vi "Test ADC command testing.vi"(8 "error in (no error)":errorcluster, 11 "TestCase in":refnum<class "Test ADC command.lvclass">) -> (0 "error out":errorcluster, 3 "TestCase out":refnum<class "Test ADC command.lvclass">)   [LabVIEW 2020, in "Test ADC command.lvclass"]
uses:
  Test ADC command.lvclass
  Implementation/Simulated Device/Simulated Device.lvclass
  <vilib>/addons/_JKI Toolkits/VI Tester/TestCase.llb/TestCase.lvclass
  C:/Program Files (x86)/National Instruments/LabVIEW 2020/vi.lib/addons/_JKI Toolkits/VI Tester/TestCase.llb/TestCase.lvclass
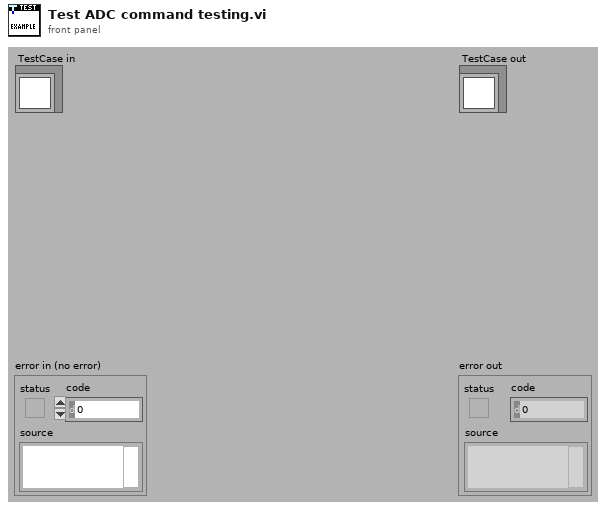
[diagram p1: front panel]
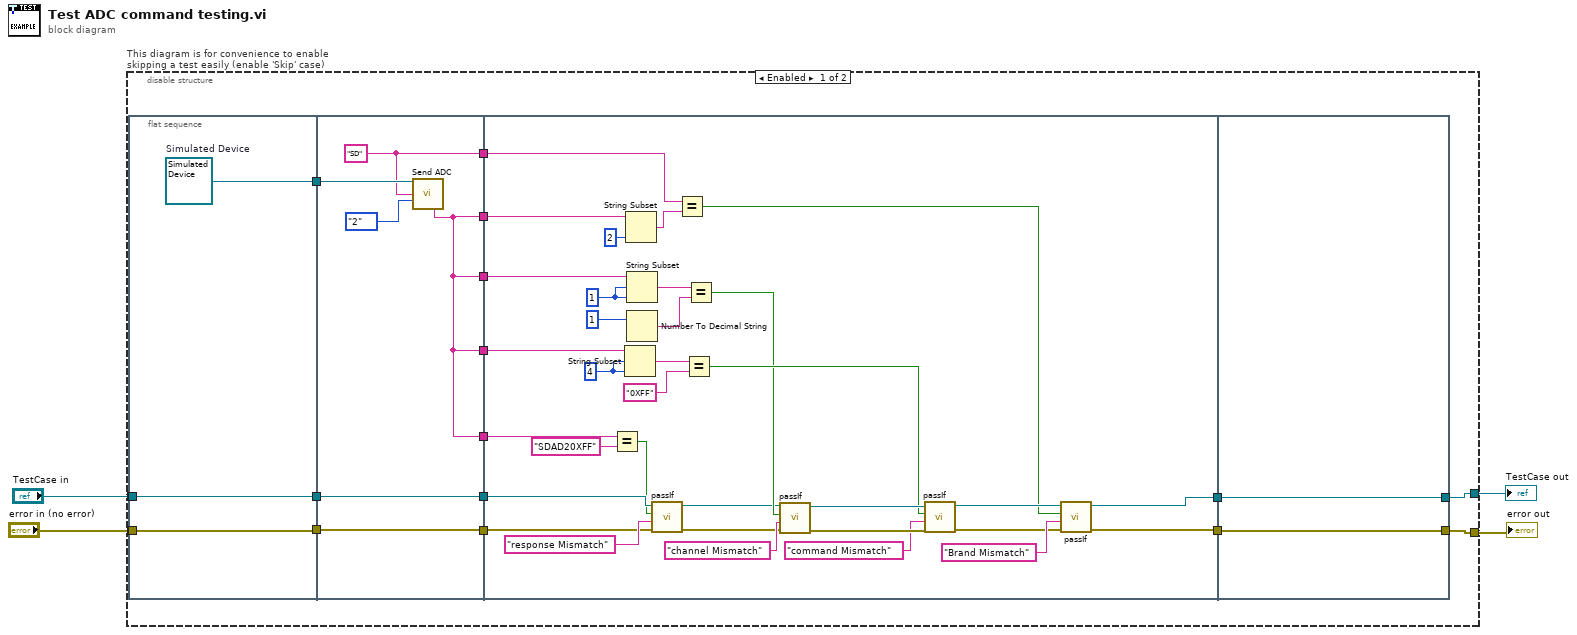
[diagram p0: block diagram]
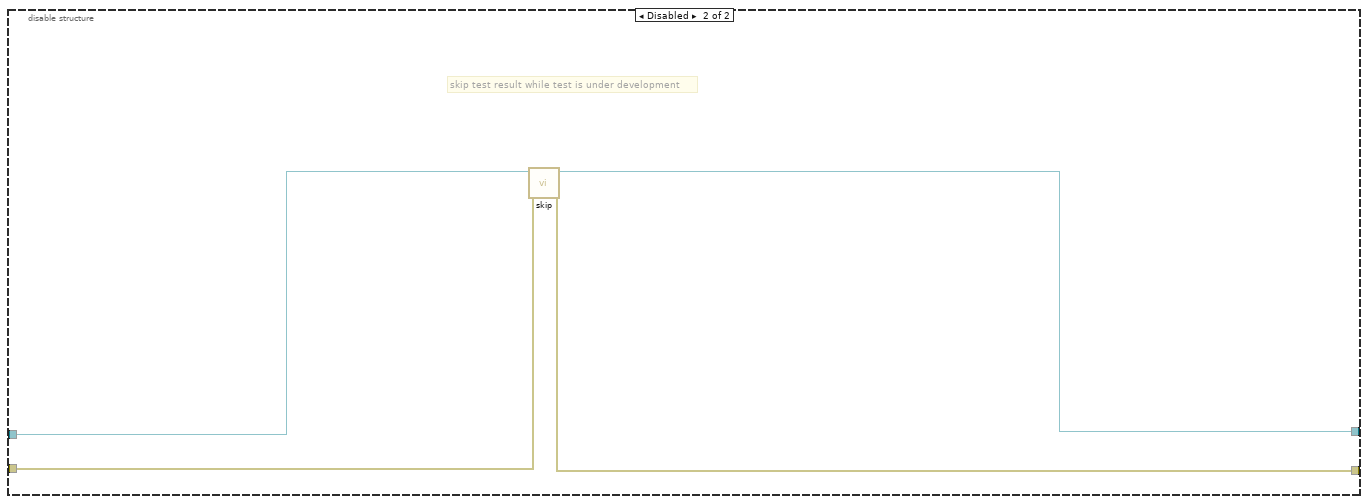
[diagram p2: hidden frame]
diagram:
  n1 = disable-structure "This diagram is for convenience to enable skipping a test easily (enable 'Skip' case)" shown="Enabled" {
    disable-tunnel: "TestCase in" -> [w19 w68]
    disable-tunnel: [w9 w66] -> w1
    disable-tunnel: [w11 w67] -> w3
    disable-tunnel: "error in (no error)" -> [w18 w65]
    frame Enabled {
      n2 = flat-sequence {
        tunnel: [w23] -> w20
        tunnel: w19 -> [w22]
        tunnel: w18 -> [w21]
        tunnel: [w22] -> w14
        tunnel: [w21] -> w12
        tunnel: w20 -> [w29]
        tunnel: [w24] -> w17
        tunnel: [w27] -> w16
        tunnel: [w26] -> w15
        tunnel: w14 -> [w26]
        tunnel: [w25] -> w13
        tunnel: w12 -> [w25]
        tunnel: [w24] -> w7
        tunnel: [w24] -> w6
        tunnel: [w24] -> w5
        tunnel: w17 -> [w61]
        tunnel: w16 -> [w60]
        tunnel: w15 -> [w34]
        tunnel: w13 -> [w32]
        tunnel: [w44] -> w10
        tunnel: [w43] -> w8
        tunnel: w7 -> [w49]
        tunnel: w6 -> [w48]
        tunnel: w5 -> [w37]
        tunnel: [w64] -> w11
        tunnel: [w63] -> w9
        tunnel: w10 -> [w63]
        tunnel: w8 -> [w64]
        frame #0 {
          w23 = refnum<class "Simulated Device.lvclass"> refnum  # Simulated Device
        }
        frame #1 {
          w27 = "SD" ("Comando")
          n3 = call-dynamic "Send ADC.vi"("Simulated Device in"=w29, "Comando"=w27, "Channel"=enum16{"2", "1"}."2") -> ("command"=w24:string)  [unwired: 8 in, 4 out]
        }
        frame #2 {
          w50 = 4 ("length (rest)")
          w57 = 1 ("length (rest)")
          n4 = Equal?(x=w37, y="SDAD20XFF") -> (x = y?=w30:bool)
          n5 = String Subset(string=w48, offset (0)=w50, length (rest)=w50) -> (substring=w51:string)
          n6 = String Subset(string=w61, length (rest)=2 ("length (rest)")) -> (substring=w58:string)  [unwired: 1 in]
          n7 = String Subset(string=w49, offset (0)=w57, length (rest)=w57) -> (substring=w56:string)
          n8 = Number To Decimal String(number=1) -> (decimal integer string=w41:string)  [unwired: 1 in]
          n9 = call-dynamic "passIf.vi"("error in (no error)"=w32, "message (\"\")"="response Mismatch" ("message (\"\")"), "pass"=w30, "TestCase in"=w34) -> ("error out"=w31:errorcluster, "TestCase out"=w33:refnum<class "Test ADC command.lvclass">)  [unwired: 6 in]
          n10 = Equal?(x=w60, y=w58) -> (x = y?=w40:bool)
          n11 = Equal?(x=w51, y="0XFF") -> (x = y?=w39:bool)
          n12 = Equal?(x=w56, y=w41) -> (x = y?=w38:bool)
          n13 = call-dynamic "passIf.vi"("error in (no error)"=w31, "message (\"\")"="channel Mismatch" ("message (\"\")"), "pass"=w38, "TestCase in"=w33) -> ("error out"=w54:errorcluster, "TestCase out"=w55:refnum<class "Test ADC command.lvclass">)  [unwired: 6 in]
          n14 = call-dynamic "passIf.vi"("error in (no error)"=w54, "message (\"\")"="command Mismatch" ("message (\"\")"), "pass"=w39, "TestCase in"=w55) -> ("error out"=w45:errorcluster, "TestCase out"=w46:refnum<class "Test ADC command.lvclass">)  [unwired: 6 in]
          n15 = call-dynamic "passIf.vi"("error in (no error)"=w45, "message (\"\")"="Brand Mismatch" ("message (\"\")"), "pass"=w40, "TestCase in"=w46) -> ("error out"=w43:errorcluster, "TestCase out"=w44:refnum<class "Test ADC command.lvclass">)  [unwired: 6 in]
        }
        frame #3 {
        }
      }
    }
    frame Disabled {
      # "skip test result while test is under development"
      n16 = call <vilib>:"skip.vi"("error in (no error)"=w65, "TestCase in"=w68) -> ("error out"=w67:errorcluster, "TestCase out"=w66:refnum<class "Test ADC command.lvclass">)  [unwired: 8 in]
    }
  }
  "error out" <- w3
  "TestCase out" <- w1
